vi "Inverter-read vi.vi"(0 "Numeric Control 6":dbl, 1 "Numeric Control 5":dbl, 2 "Numeric Control 4":dbl, 3 "Numeric Control 16":dbl, 4 "Numeric Control 15":dbl, 6 "Numeric Control 17":u32, 7 "Numeric Control 14":dbl, 8 "register values":u16[](array[numeric]), 9 "Numeric Control 13":dbl, 11 "Numeric Control 12":dbl) -> (10 "Numeric Control 3":dbl, 12 "Numeric Control 2":dbl, 13 "Numeric Control 7":dbl, 14 "Numeric Control":dbl, 15 "Numeric Control 10":dbl, 16 "Numeric Control 11":dbl, 17 "Numeric Control 9":dbl, 18 "Numeric Control 8":dbl)   [LabVIEW 2016]
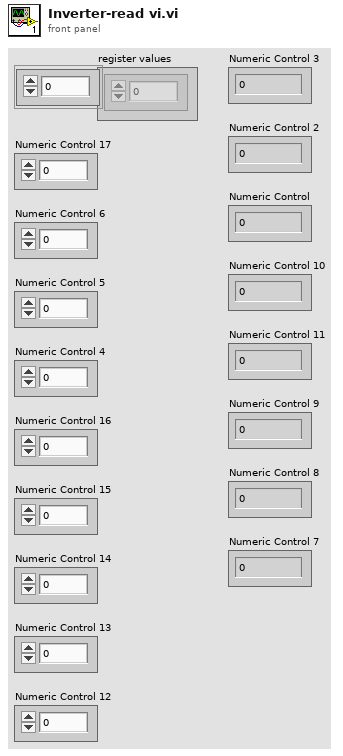
[diagram p1: front panel]
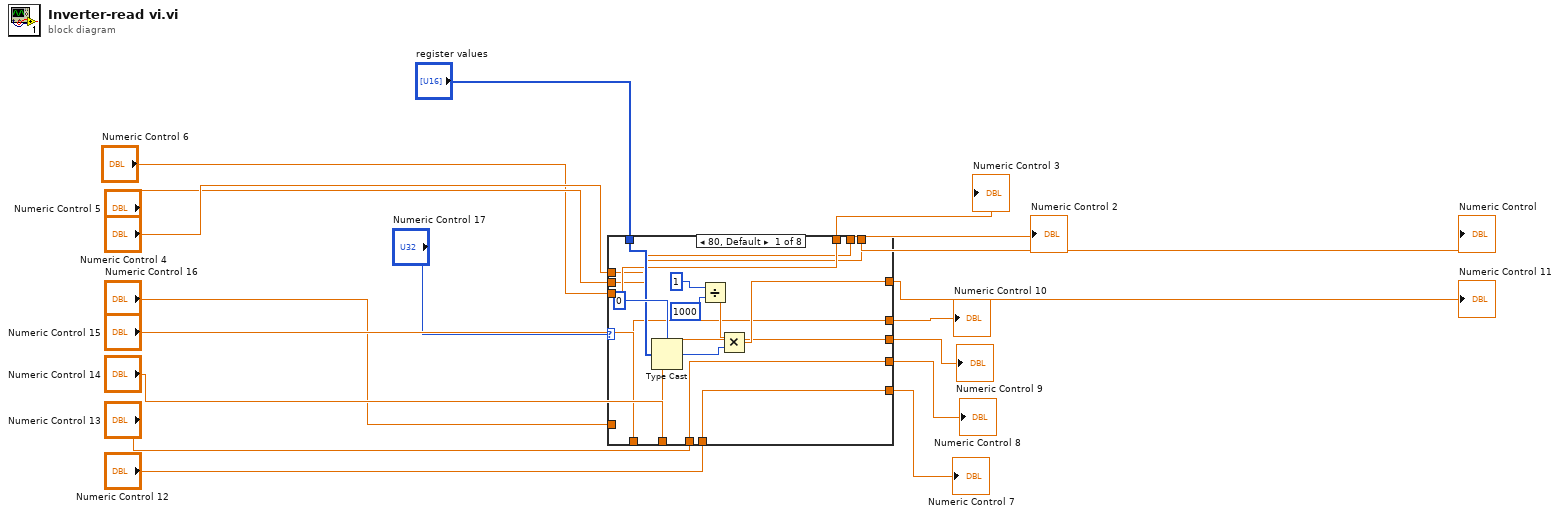
[diagram p0: block diagram]
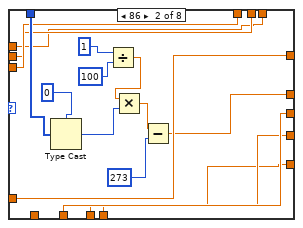
[diagram p2: hidden frame]
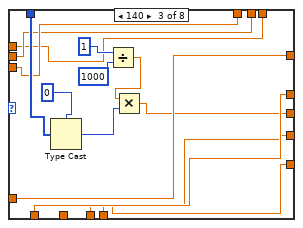
[diagram p3: hidden frame]
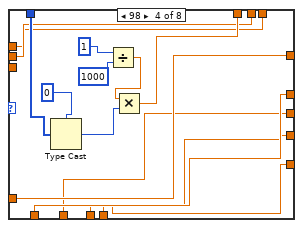
[diagram p4: hidden frame]
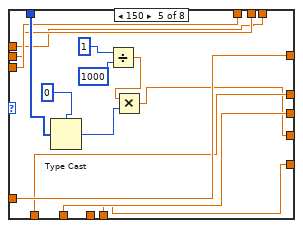
[diagram p5: hidden frame]
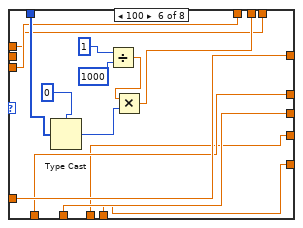
[diagram p6: hidden frame]
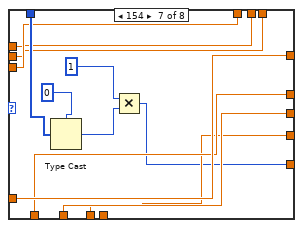
[diagram p7: hidden frame]
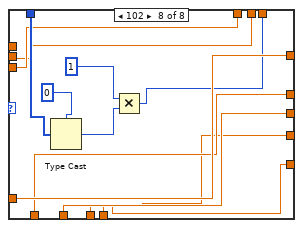
[diagram p8: hidden frame]
diagram:
  n1 = case shown="80, Default" "Numeric Control 17" {
    tunnel: "register values" -> [w27 w39 w56 w70 w84 w98 w113 w125]
    tunnel: [w26 w43 w59 w73 w87 w101 w116 w128] -> w8
    tunnel: "Numeric Control 16" -> [_ w43 w59 w73 w87 w101 w116 w128]
    tunnel: [w25 w42 w55 w69 w83 w97 w112 w124] -> w9
    tunnel: "Numeric Control 15" -> [w25 _ w55 w69 w83 w97 w112 w124]
    tunnel: [w24 w38 w54 w66 w82 w96 w111 w123] -> w10
    tunnel: "Numeric Control 14" -> [w24 w38 _ w66 w82 w96 w111 w123]
    tunnel: [w23 w37 w53 w68 w81 w93 w110 w122] -> w11
    tunnel: "Numeric Control 13" -> [w23 w37 w53 w68 _ w93 w110 w122]
    tunnel: [w22 w36 w52 w67 w80 w95 w109 w118] -> w12
    tunnel: "Numeric Control 12" -> [w22 w36 w52 w67 w80 w95 _ w118]
    tunnel: [w21 w35 w51 w65 w79 w94 w107 w120] -> w16
    tunnel: "Numeric Control 6" -> [w21 w35 w51 _ w79 w94 w107 w120]
    tunnel: [w20 w34 w50 w64 w78 w92 w106 w119] -> w17
    tunnel: "Numeric Control 5" -> [w20 w34 w50 w64 w78 _ w106 w119]
    tunnel: [w19 w33 w49 w63 w77 w91 w105 w117] -> w18
    tunnel: "Numeric Control 4" -> [w19 w33 w49 w63 w77 w91 w105 _]
    frame 80, Default {
      n2 = Type Cast(type=u32 0, x=w27) -> (*(type *) &x=w31:u32)
      n3 = Divide(x=u32 1, y=u32 1000) -> (x/y=w28:dbl)
      n4 = Multiply(x=w28, y=w31) -> (x*y=w26:dbl)
    }
    frame 86 {
      n5 = Type Cast(type=u16 0, x=w39) -> (*(type *) &x=w41:u16)
      n6 = Divide(x=u32 1, y=u32 100) -> (x/y=w45:dbl)
      n7 = Multiply(x=w45, y=w41) -> (x*y=w44:dbl)
      n8 = Subtract(x=w44, y=273) -> (x-y=w42:dbl)
    }
    frame 140 {
      n9 = Type Cast(type=u32 0, x=w56) -> (*(type *) &x=w58:u32)
      n10 = Divide(x=u32 1, y=u32 1000) -> (x/y=w60:dbl)
      n11 = Multiply(x=w60, y=w58) -> (x*y=w54:dbl)
    }
    frame 98 {
      n12 = Type Cast(type=u32 0, x=w70) -> (*(type *) &x=w72:u32)
      n13 = Divide(x=u32 1, y=u32 1000) -> (x/y=w74:dbl)
      n14 = Multiply(x=w74, y=w72) -> (x*y=w65:dbl)
    }
    frame 150 {
      n15 = Type Cast(type=0, x=w84) -> (*(type *) &x=w86:i32)
      n16 = Divide(x=u32 1, y=u32 1000) -> (x/y=w88:dbl)
      n17 = Multiply(x=w88, y=w86) -> (x*y=w81:dbl)
    }
    frame 100 {
      n18 = Type Cast(type=0, x=w98) -> (*(type *) &x=w100:i32)
      n19 = Divide(x=u32 1, y=u32 1000) -> (x/y=w102:dbl)
      n20 = Multiply(x=w102, y=w100) -> (x*y=w92:dbl)
    }
    frame 154 {
      n21 = Type Cast(type=0, x=w113) -> (*(type *) &x=w115:i32)
      n22 = Multiply(x=1, y=w115) -> (x*y=w109:i32)
    }
    frame 102 {
      n23 = Type Cast(type=0, x=w125) -> (*(type *) &x=w127:i32)
      n24 = Multiply(x=1, y=w127) -> (x*y=w117:i32)
    }
  }
  "Numeric Control" <- w18
  "Numeric Control 2" <- w17
  "Numeric Control 3" <- w16
  "Numeric Control 7" <- w12
  "Numeric Control 8" <- w11
  "Numeric Control 9" <- w10
  "Numeric Control 10" <- w9
  "Numeric Control 11" <- w8
